vi "write TBM configuration.vi"(8 "error in":errorcluster, 10 "configuration":refnum<class "TBM configuration.lvclass">, 11 "Modbus Slave editor node in":refnum<class "Modbus Slave editor node.lvclass">) -> (0 "error out":errorcluster, 3 "Modbus Slave editor node out":refnum<class "Modbus Slave editor node.lvclass">)   [LabVIEW 2013, in "Modbus Slave editor node.lvclass"]
doc: "Platypus Framework 1.0.1.65\nNI Systems Engineering - National Instruments"
uses:
  Modbus Slave editor node.lvclass
  <vilib>/NI/Tag Bus Module Framework/root configuration/TBM configuration.lvclass
  <vilib>/NI/TBM Modules/modbus slave/configuration/Modbus Slave configuration.lvclass
  Modbus Slave editor node.lvclass/Modbus Slave editor node.ctl
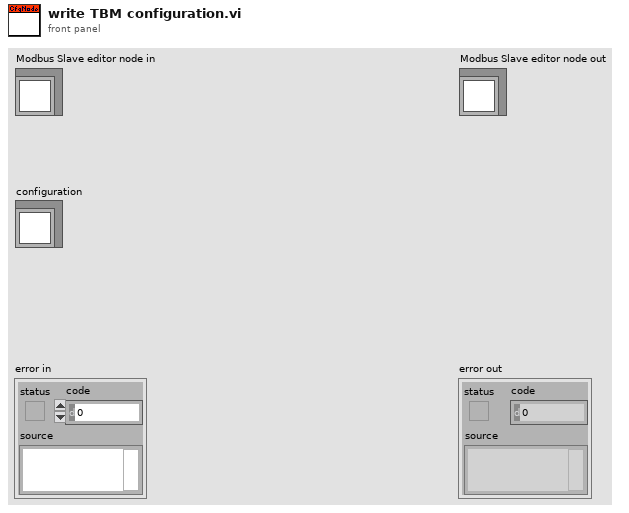
[diagram p1: front panel]
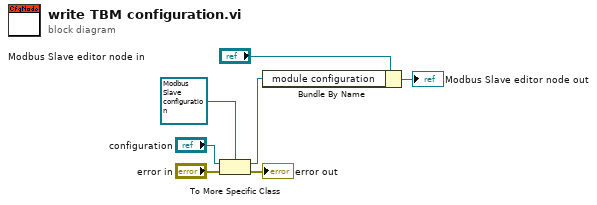
[diagram p0: block diagram]
diagram:
  n1 = To More Specific Class(target class=refnum<class "Modbus Slave configuration.lvclass"> refnum ("module configuration"), reference="configuration", error in="error in") -> (specific class reference=w1:refnum<class "Modbus Slave configuration.lvclass">, error out=→"error out":errorcluster)
  n2 = Bundle By Name(cluster="Modbus Slave editor node in", "module configuration"=w1) -> (→"Modbus Slave editor node out":refnum<class "Modbus Slave editor node.lvclass">)
